vi "Close HVPS.vi"(8 "error in":errorcluster, 11 "SR 3XX HVPS in":refnum<class "SR 3XX HVPS.lvclass">) -> (0 "error out":errorcluster, 3 "SR 3XX HVPS out":refnum<class "SR 3XX HVPS.lvclass">)   [LabVIEW 2014, in "SR 3XX HVPS.lvclass"]
doc: "Close the GPIB connection to the power supply."
uses:
  SR 3XX HVPS.lvclass
  SR 3XX HVPS.lvclass/SR 3XX HVPS.ctl
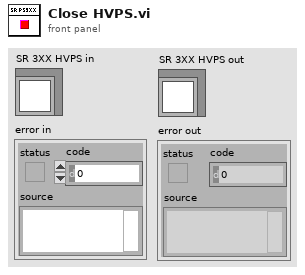
[diagram p1: front panel]
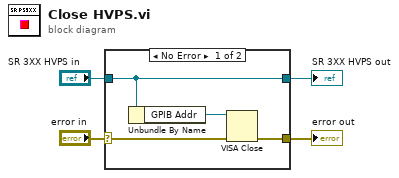
[diagram p0: block diagram]
diagram:
  n1 = case shown="No Error" "error in" {
    selector: "error in" -> [w6 w10]
    tunnel: [w5 w10] -> w3
    tunnel: [w8 w9] -> w1
    tunnel: "SR 3XX HVPS in" -> [w8 w9]
    frame No Error {
      n2 = Unbundle By Name(w8) -> ("GPIB Addr"=w7:refnum<visa-resource-name>)
      n3 = VISA Close(VISA resource name=w7, error in (no error)=w6) -> (error out=w5:errorcluster)
    }
    frame Error {
    }
  }
  "error out" <- w3
  "SR 3XX HVPS out" <- w1
